vi "Set Intensity Graph Cursor.vi"(8 "error in (no error)":errorcluster, 10 "Cursor.Cursor Position":T1, 11 "graph_utilities in":refnum<class "graph_utilities.lvclass">) -> (0 "error out":errorcluster, 3 "graph_utilities out":refnum<class "graph_utilities.lvclass">)   [LabVIEW 2019, in "graph_utilities.lvclass"]
doc: "Set the cursor position on the Intensity Graph"
uses:
  graph_utilities.lvclass
  <vilib>/Utility/miscctls.llb/LVPointDoubleTypeDef.ctl
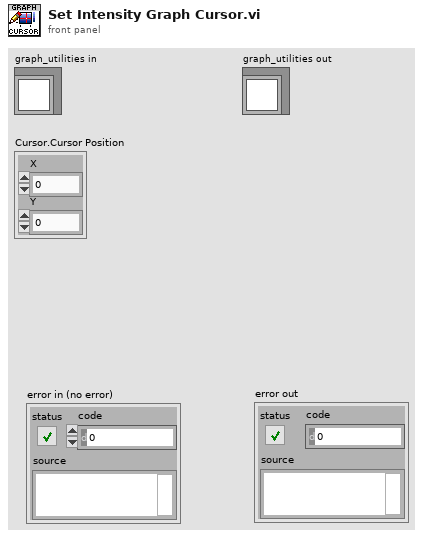
[diagram p1: front panel]
types:
  T1 = typedef "LVPointDoubleTypeDef.ctl" = cluster{"X":dbl, "Y":dbl}
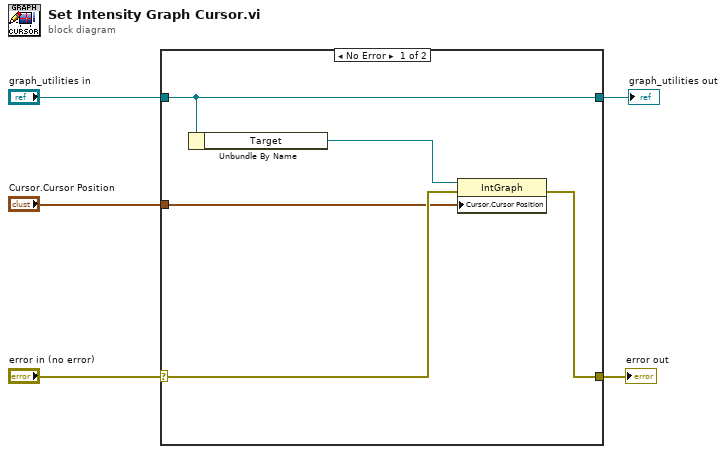
[diagram p0: block diagram]
diagram:
  n1 = case shown="No Error" "error in (no error)" {
    selector: "error in (no error)" -> [w9 w12]
    tunnel: "Cursor.Cursor Position" -> [w6 _]
    tunnel: [w10 w12] -> w4
    tunnel: "graph_utilities in" -> [w8 w11]
    tunnel: [w8 w11] -> w1
    frame No Error {
      n2 = Unbundle By Name(w8) -> ("Target"=w7:refnum<vi>)
      n3 = property on="Property Node" class="IntGraph"(reference=w7, error in=w9, "Cursor.Cursor Position"=w6) -> (error out=w10:errorcluster)  [unwired: 1 out]
    }
    frame Error {
    }
  }
  "error out" <- w4
  "graph_utilities out" <- w1
